vi "GE 5565PIORC.Pointer.New.vi"(8 "error in (no error)":errorcluster, 11 "size in bytes":u32) -> (0 "error out":errorcluster, 3 "pointer":u64 format="%08x")   [LabVIEW 2016, in "GE 5565PIORC.lvclass"]
doc: "Allocates a new pointer using the LabVIEW Memory Manager. The pointer will point to a block of memory of length <b>size in bytes</b>."
uses:
  GE 5565PIORC.lvclass
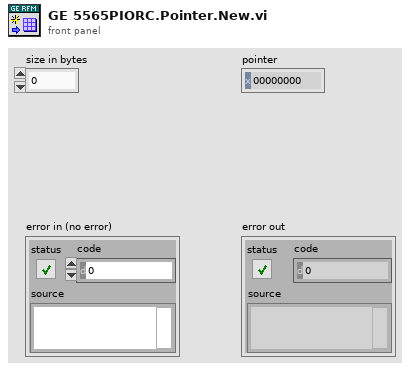
[diagram p1: front panel]
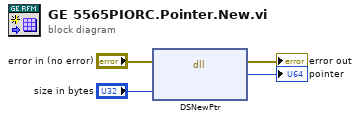
[diagram p0: block diagram]
diagram:
  n1 = dll-call lib="LabVIEW" fn="DSNewPtr"(error in="error in (no error)", "size"="size in bytes") -> (error out=→"error out":errorcluster, "pointer"=→"pointer":u64)  [unwired: 3 in, 1 out]
